vi "과제5.vi"() -> ()   [LabVIEW 2013]
panel:
  in  "A":dbl
  in  "B":dbl
  out "결과":dbl
  in  "+":bool
  in  "-":bool
  in  "/":bool
  in  "*":bool
  in  "정지":bool
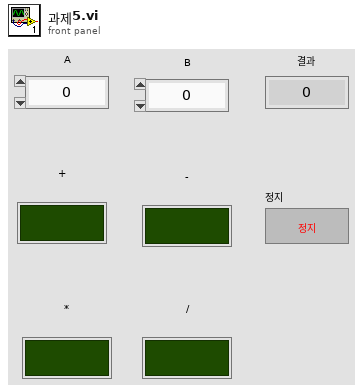
[diagram p1: front panel]
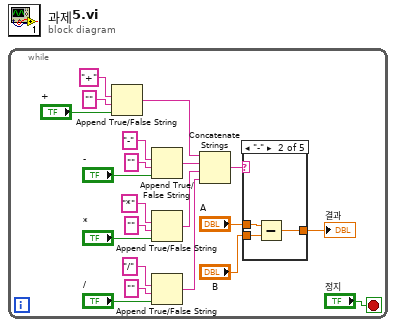
[diagram p0: block diagram]
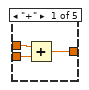
[diagram p2: hidden frame]
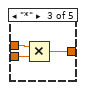
[diagram p3: hidden frame]
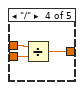
[diagram p4: hidden frame]
diagram:
  n1 = while {
    stop <- "정지" stop-if-true
    n2 = Append True/False String(1:"+", 2:"" ("참 문자열"), 3:"+" ("문자열(\"\")")) -> (0:w17:string)  [unwired: 1 in]
    n3 = Append True/False String(1:"-", 2:"" ("참 문자열"), 3:"-" ("문자열(\"\")")) -> (0:w16:string)  [unwired: 1 in]
    n4 = Append True/False String(1:"*", 2:"" ("참 문자열"), 3:"*" ("문자열(\"\")")) -> (0:w14:string)  [unwired: 1 in]
    n5 = Append True/False String(1:"/", 2:"" ("참 문자열"), 3:"/" ("문자열(\"\")")) -> (0:w15:string)  [unwired: 1 in]
    n6 = Concatenate Strings(w17, w16, w14, w15) -> (w18:string)
    n7 = case shown="\"-\"" w18 {
      tunnel: "A" -> [w24 w27 w30 w33 _]
      tunnel: "B" -> [w23 w26 w29 w32 _]
      tunnel: [w22 w25 w28 w31 _] -> w19
      frame "+" {
        n8 = Add(x=w24, y=w23) -> (x+y=w22:dbl)
      }
      frame "-" {
        n9 = Subtract(x=w27, y=w26) -> (x-y=w25:dbl)
      }
      frame "*" {
        n10 = Multiply(x=w30, y=w29) -> (x*y=w28:dbl)
      }
      frame "/" {
        n11 = Divide(x=w33, y=w32) -> (x/y=w31:dbl)
      }
      frame Default {
      }
    }
    "결과" <- w19
  }
